vi "Split Lines.vi"(10 "String In":string) -> (2 "Lines Out":string[](array[string]))   [LabVIEW 2017]
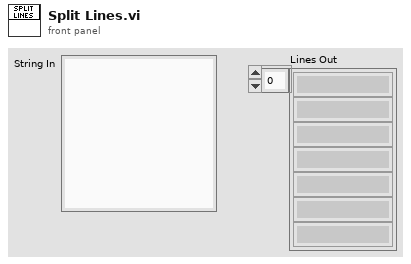
[diagram p1: front panel]
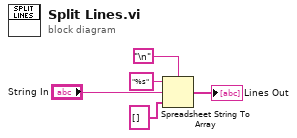
[diagram p0: block diagram]
diagram:
  n1 = Spreadsheet String To Array(delimiter (Tab)="\n", format string="%s", spreadsheet string="String In", array type (2D Dbl)=string[] [] ("Lines Out 2")) -> (array=→"Lines Out":string[])
